vi "Test_Grid.vi"() -> ()   [LabVIEW 2020]
panel:
  in  "Draw Center":bool
  in  "Horiz step":i32=1 min=1 max=10000 step=1
  in  "Clear Overlay":bool
  in  "Vertical step":i32=1 min=1 max=10000 step=1
  in  "Color":u32(colorbox)=16711680
  in  "Draw Grid":bool
  in  "stop":bool
  out "Image":T1(plugin-control)
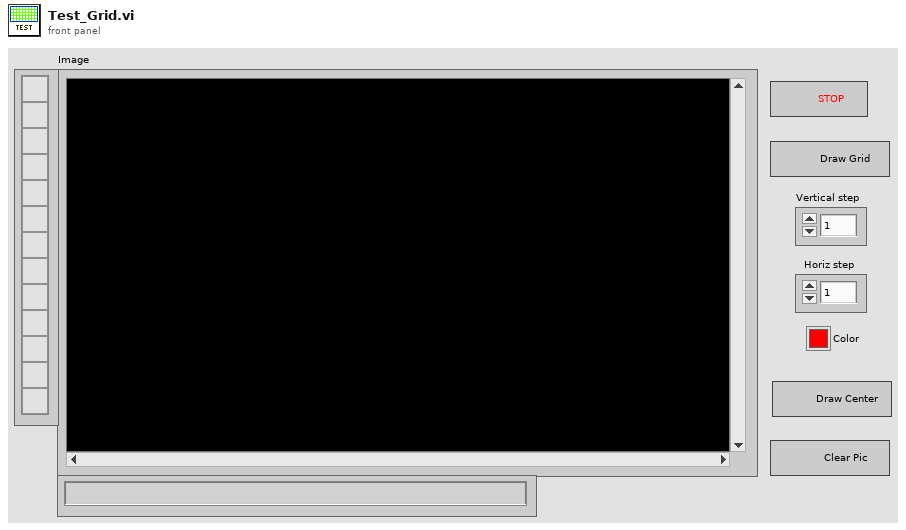
[diagram p1: front panel]
types:
  T1 = typedef "IMAQ Image.ctl" = refnum<image>
  T2 = typedef "Image Type" = u32
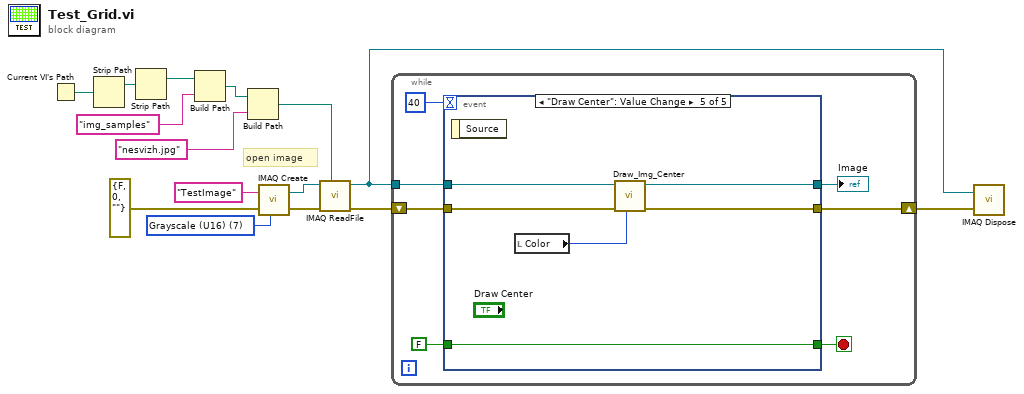
[diagram p0: block diagram]
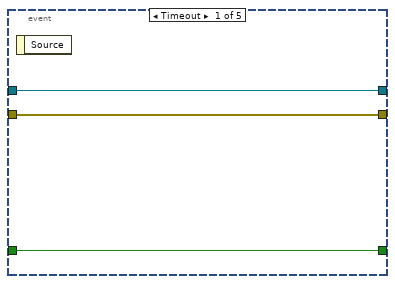
[diagram p2: hidden frame]
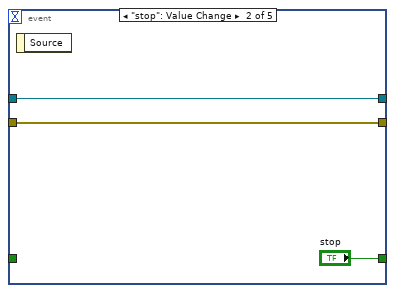
[diagram p3: hidden frame]
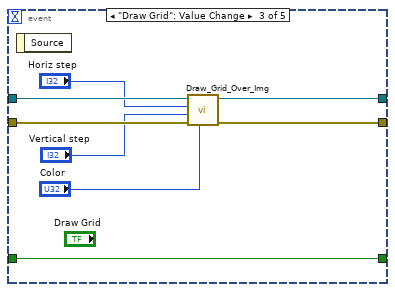
[diagram p4: hidden frame]
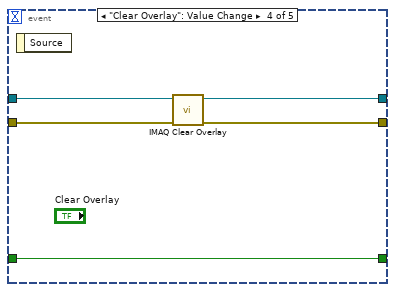
[diagram p5: hidden frame]
diagram:
  w11 = T2 7 items=["Grayscale (U8)", "Grayscale (I16)", "Grayscale (SGL)", "Complex (CSG)", "RGB (U32)", "HSL (U32)", "RGB (U64)", "Grayscale (U16)"] ("Image Type")
  # "open image"
  n1 = Current VI's Path() -> (path=w15:path)
  n2 = Strip Path(path=w15) -> (stripped path=w7:path)  [unwired: 1 out]
  n3 = Strip Path(path=w7) -> (stripped path=w6:path)  [unwired: 1 out]
  n4 = Build Path(base path=w6, name or relative path="img_samples") -> (appended path=w4:path)
  n5 = Build Path(base path=w4, name or relative path="nesvizh.jpg") -> (appended path=w13:path)
  n6 = call "IMAQ Create"("Image Name"="TestImage", "Image Type"=w11, "error in (no error)"=errorcluster {"status"=FALSE, "code"=0, "source"=""}) -> ("New Image"=w9:T1, "error out"=w10:errorcluster)  [unwired: 2 in]
  n7 = call "IMAQ ReadFile"("File Path"=w13, "error in (no error)"=w10, "Image"=w9) -> ("error out"=w3:errorcluster, "Image Out"=w1:T1)  [unwired: 4 in, 3 out]
  n8 = while {
    shift-right: [w20] -> w2
    shift-left: w3 -> [w21]
    tunnel: w1 -> [w19]
    stop <- w16 stop-if-true
    n9 = event shown="[4] \"Draw Center\": Value Change" {
      selector: _ -> [_ _ _ _ _]
      dyn-events: _ -> [_ _ _ _ _]
      timeout: 40 -> [_ _ _ _ _]
      tunnel: w21 -> [w24 w28 w36 w40 w46]
      tunnel: [w24 w28 w32 w38 w44] -> w20
      tunnel: [w23 "stop" w31 w41 w47] -> w16
      tunnel: w19 -> [w25 w26 w34 w39 w45]
      tunnel: [w25 w26 w33 w37 w43] -> w18
      tunnel: FALSE ("stop") -> [w23 _ w31 w41 w47]
      event Timeout {
        n10 = event-data() -> ()  [unwired: 1 in, 1 out]
      }
      event "stop": Value Change {
        n11 = event-data() -> ()  [unwired: 1 in, 1 out]
      }
      event "Draw Grid": Value Change {
        n12 = event-data() -> ()  [unwired: 1 in, 1 out]
        n13 = call "Draw_Grid_Over_Img.vi"("[IN] Color"="Color", "error IN"=w36, "[IN] Vertical step"="Vertical step", "[IN] Horiz step"="Horiz step", "[IN] Image"=w34) -> ("error OUT"=w32:errorcluster, "[OUT] Image"=w33:T1)  [unwired: 5 in]
      }
      event "Clear Overlay": Value Change {
        n14 = event-data() -> ()  [unwired: 1 in, 1 out]
        n15 = call "IMAQ Clear Overlay"("error in (no error)"=w40, "Image"=w39) -> ("error out"=w38:errorcluster, "Image Out"=w37:T1)  [unwired: 8 in]
      }
      event "Draw Center": Value Change {
        n16 = event-data() -> ()  [unwired: 1 in, 1 out]
        n17 = local read "Color"() -> (w42:u32)
        n18 = call "Draw_Img_Center.vi"("[IN] Color"=w42, "error IN"=w46, "[IN] Image"=w45) -> ("error OUT"=w44:errorcluster, "[OUT] Image"=w43:T1)  [unwired: 7 in]
      }
    }
    "Image" <- w18
  }
  n19 = call "IMAQ Dispose"("Image"=w1, "error in (no error)"=w2) -> ()  [unwired: 4 in, 1 out]
